vi "initialise_coolprop.vi"(8 "error in (no error)":errorcluster, 9 "Path to CoolProp.dll":path=path "C:/Labview/Libfolder/CoolProp.dll", 10 "FluidOfInterest":T3="Water") -> (0 "error out":errorcluster, 2 "Fluid Data":T2, 3 "Common Out":T1)   [LabVIEW 2017]
doc: "VI used to initialise fluid data clusters.\nUses type defined controls as in/output (included in the library):\n-FluidOfInterest.ctl - contains a full list of all possible fluids\n-FluidCommon.ctl - Common output cluster required in calculate_coolprop.vi\n-FluidData.ctl - Cluster containing fluid properties values\n\n---\nDesigned by Department of Industrial System and Product Design, Ghent University.\nContact: sergei.gusev@ugent.be; jan.nolens@ugent.be\n\nBased on a Labview-Refprop Wrapper downloaded from Nist.org\nMore info: ken_pop@tom.com yan.ding@jci.com"
uses:
  FluidOfInterest.ctl
  FluidData.ctl
  FluidCommon.ctl
panel:
  in  "Common In":T1
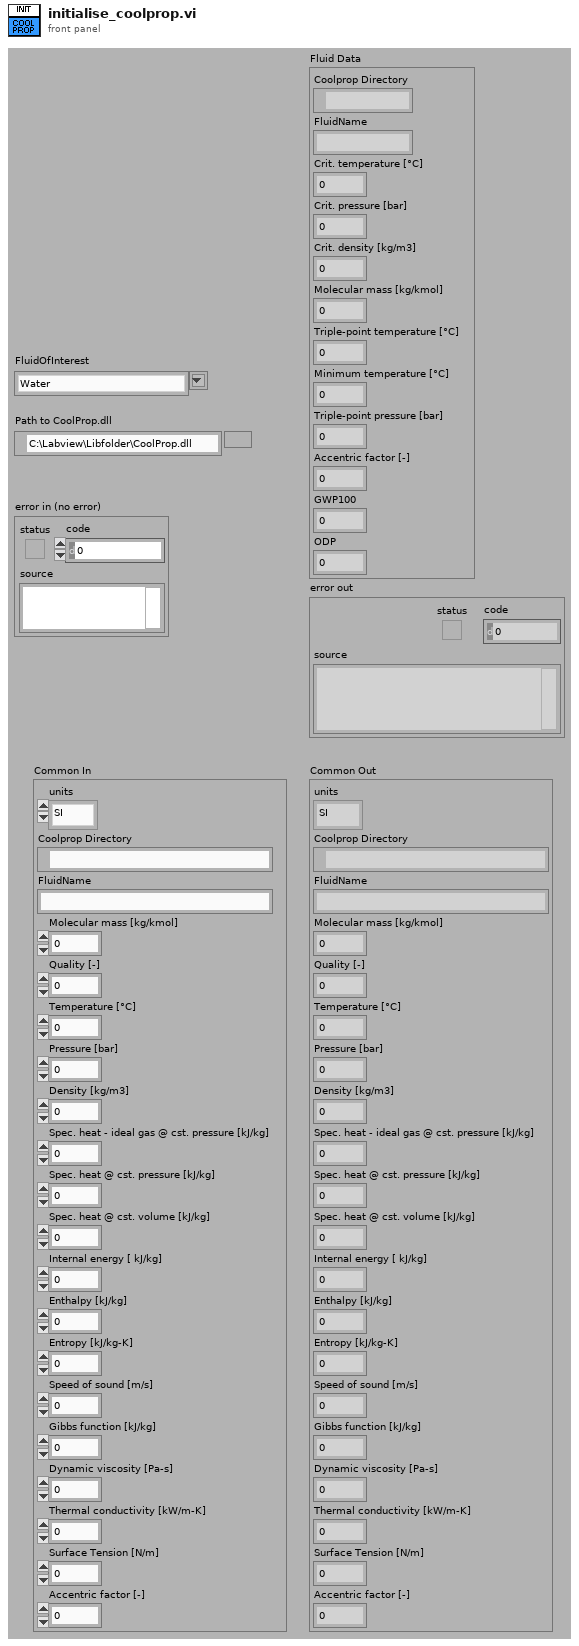
[diagram p1: front panel]
types:
  T1 = typedef "FluidCommon.ctl" = cluster{"units":enum16{"SI", "IP"}, "Coolprop Directory":path, "FluidName":string, "Molecular mass [kg/kmol]":dbl, "Quality [-]":dbl, "Temperature [°C]":dbl, "Pressure [bar]":dbl, "Density [kg/m3]":dbl, "Spec. heat - ideal gas @ cst. pressure [kJ/kg]":dbl, "Spec. heat @ cst. pressure [kJ/kg]":dbl, "Spec. heat @ cst. volume [kJ/kg]":dbl, "Internal energy [ kJ/kg]":dbl, "Enthalpy [kJ/kg]":dbl, "Entropy [kJ/kg-K]":dbl, "Speed of sound [m/s]":dbl, "Gibbs function [kJ/kg]":dbl, "Dynamic viscosity [Pa-s]":dbl, "Thermal conductivity [kW/m-K]":dbl, "Surface Tension [N/m]":dbl, "Accentric factor [-]":dbl}
  T2 = typedef "FluidData.ctl" = cluster{"Coolprop Directory":path, "FluidName":string, "Crit. temperature [°C]":dbl, "Crit. pressure [bar]":dbl, "Crit. density [kg/m3]":dbl, "Molecular mass [kg/kmol]":dbl, "Triple-point temperature [°C]":dbl, "Minimum temperature [°C]":dbl, "Triple-point pressure [bar]":dbl, "Accentric factor [-]":dbl, "GWP100":dbl, "ODP":dbl}
  T3 = typedef "FluidOfInterest.ctl" = string
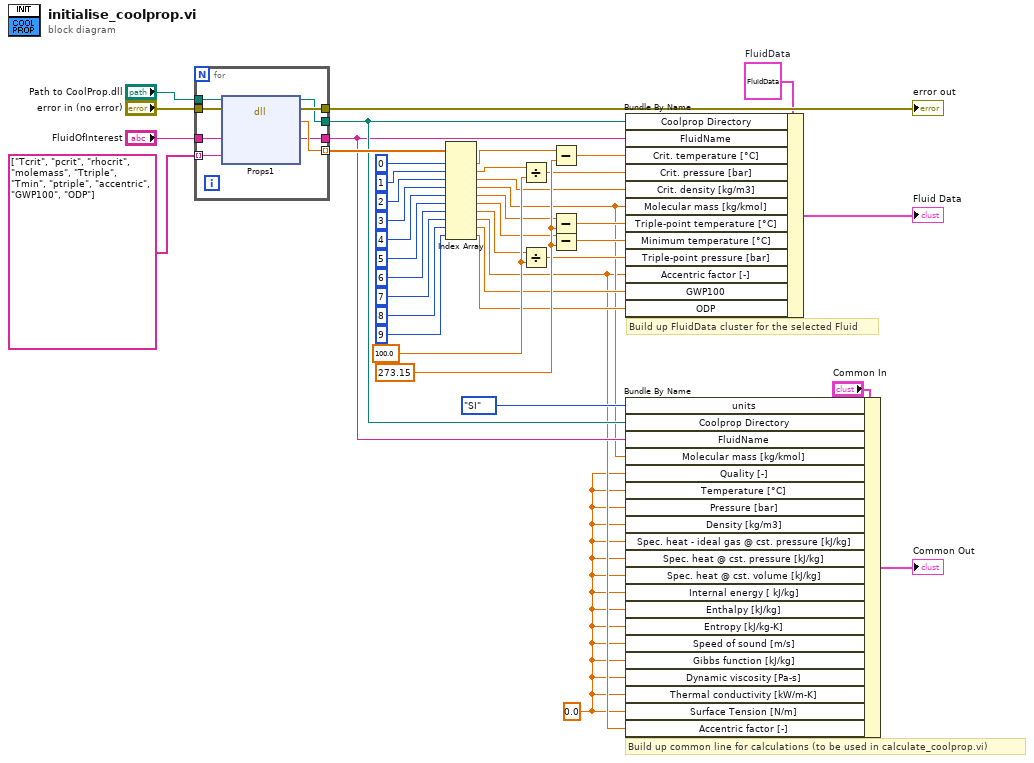
[diagram p0: block diagram]
diagram:
  w1 = 0.0 ("Surface Tension [N/m]")
  w18 = 100.0
  w22 = 273.15
  w37 = T2 {"Coolprop Directory"=path "", "FluidName"="", "Crit. temperature [°C]"=0.0, "Crit. pressure [bar]"=0.0, "Crit. density [kg/m3]"=0.0, "Molecular mass [kg/kmol]"=0.0, "Triple-point temperature [°C]"=0.0, "Minimum temperature [°C]"=0.0, "Triple-point pressure [bar]"=0.0, "Accentric factor [-]"=0.0, "GWP100"=0.0, "ODP"=0.0}  # FluidData
  # "Build up FluidData cluster for the selected Fluid"
  # "Build up common line for calculations (to be used in calculate_coolprop.vi)"
  n1 = for {
    tunnel: "FluidOfInterest" -> [w49]
    tunnel: "Path to CoolProp.dll" -> [w48]
    tunnel: string[] ["Tcrit", "pcrit", "rhocrit", "molemass", "Ttriple", "Tmin", "ptriple", "accentric", "GWP100", "ODP"] ("Array") -> [w44] mode=indexing
    tunnel: [w45] -> w36 mode=indexing
    tunnel: "error in (no error)" -> [w47]
    tunnel: [w46] -> w38
    tunnel: [w43] -> w4
    tunnel: [w42] -> w5
    n2 = dll-call lib="C:/Users/jan.nolens/Desktop/CoolProp.dll" fn="Props1"(path in=w48, error in=w47, "Fluid"=w49, "PropName"=w44) -> (path out=w42:path, error out=w46:errorcluster, "OutputValue"=w45:dbl, "Fluid"=w43:string)  [unwired: 1 in, 1 out]
  }
  "error out" <- w38
  n3 = Index Array(array=w36, index #1=0 ("index"), index #2=1 ("index"), index #3=2 ("index"), index #4=3 ("index"), index #5=4 ("index"), index #6=5 ("index"), index #7=6 ("index"), index #8=7 ("index"), index #9=8 ("index"), index #10=9 ("index")) -> (element #1=w21:dbl, element #2=w17:dbl, element #3=w16:dbl, element #4=w3:dbl, element #5=w15:dbl, element #6=w14:dbl, element #7=w13:dbl, element #8=w2:dbl, element #9=w12:dbl, element #10=w11:dbl)
  n4 = Divide(x=w17, y=w18) -> (x/y=w20:dbl)
  n5 = Divide(x=w13, y=w18) -> (x/y=w19:dbl)
  n6 = Subtract(x=w21, y=w22) -> (x-y=w25:dbl)
  n7 = Subtract(x=w15, y=w22) -> (x-y=w24:dbl)
  n8 = Subtract(x=w14, y=w22) -> (x-y=w23:dbl)
  n9 = Bundle By Name(cluster=w37, "Coolprop Directory"=w5, "FluidName"=w4, "Crit. temperature [°C]"=w25, "Crit. pressure [bar]"=w20, "Crit. density [kg/m3]"=w16, "Molecular mass [kg/kmol]"=w3, "Triple-point temperature [°C]"=w24, "Minimum temperature [°C]"=w23, "Triple-point pressure [bar]"=w19, "Accentric factor [-]"=w2, "GWP100"=w12, "ODP"=w11) -> (→"Fluid Data":T2)
  n10 = Bundle By Name(cluster="Common In", "units"=enum16{"SI", "IP"}."SI", "Coolprop Directory"=w5, "FluidName"=w4, "Molecular mass [kg/kmol]"=w3, "Quality [-]"=w1, "Temperature [°C]"=w1, "Pressure [bar]"=w1, "Density [kg/m3]"=w1, "Spec. heat - ideal gas @ cst. pressure [kJ/kg]"=w1, "Spec. heat @ cst. pressure [kJ/kg]"=w1, "Spec. heat @ cst. volume [kJ/kg]"=w1, "Internal energy [ kJ/kg]"=w1, "Enthalpy [kJ/kg]"=w1, "Entropy [kJ/kg-K]"=w1, "Speed of sound [m/s]"=w1, "Gibbs function [kJ/kg]"=w1, "Dynamic viscosity [Pa-s]"=w1, "Thermal conductivity [kW/m-K]"=w1, "Surface Tension [N/m]"=w1, "Accentric factor [-]"=w2) -> (→"Common Out":T1)
